vi "String to Boolean.vi"() -> ()   [LabVIEW 2017]
panel:
  in  "y":bool
  in  "x":bool
  out "BLAH BLAH":bool
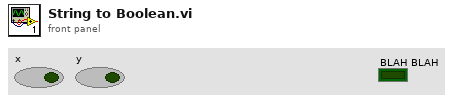
[diagram p1: front panel]
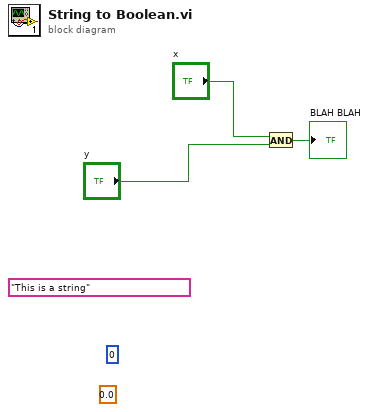
[diagram p0: block diagram]
diagram:
  (unwired) 0.0
  (unwired) 0
  (unwired) "This is a string"
  n1 = And(x="x", y="y") -> (x .and. y?=→"BLAH BLAH":bool)
